vi "Requests.vi"(8 "error in (no error)":errorcluster, 9 "write enable":bool=TRUE, 11 "Serial in":refnum<class "Serial.lvclass">) -> (0 "error out":errorcluster, 3 "Serial out":refnum<class "Serial.lvclass">)   [LabVIEW 2021, in "Serial.lvclass"]
uses:
  Serial.lvclass
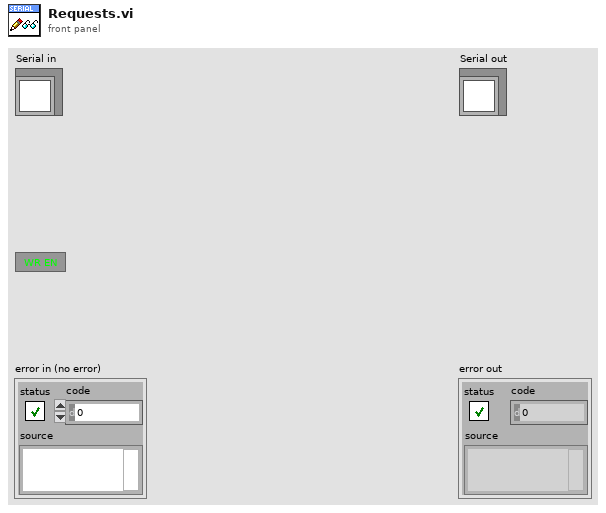
[diagram p1: front panel]
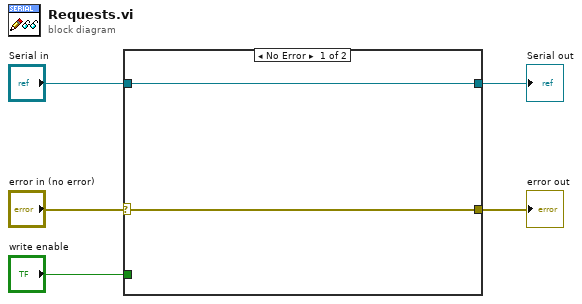
[diagram p0: block diagram]
diagram:
  n1 = case shown="No Error" "error in (no error)" {
    selector: "error in (no error)" -> [w6 w9]
    tunnel: [w6 w9] -> w3
    tunnel: [w7 w8] -> w4
    tunnel: "Serial in" -> [w7 w8]
    tunnel: "write enable" -> [_ _]
    frame No Error {
    }
    frame Error {
    }
  }
  "error out" <- w3
  "Serial out" <- w4
